vi "graphModule.vi"() -> ()   [LabVIEW 2023]
uses:
  <vilib>/Utility/miscctls.llb/LVCursorListTypeDef.ctl
panel:
  in  "Linked?":bool
  out "gate":i32
  out "Cursor Out":dbl[](array[numeric])=[128.0, 112.0, 144.0, 96.0, 160.0]
  in  "Cursor List":T1=[{"Name"="FGV", "Color"=99999, "Style"=2, "Point Style"=0, "Name Visible"=FALSE, "Allow Drag"=TRUE, "Cursor Mode"=1, "Plot"=0, "Index"=128, "Position"={"X"=128.0, "Y"=0.0}, "X Scale"=0, "Y Scale"=0, "Watch Plots"=[], "Watch All Plots"=FALSE, "Plot Area"=0, "Label Offset"={"X"=0.0, "Y"=0.0}}, {"Name"="Lower Bound", "Color"=50000, "Style"=2, "Point Style"=0, "Name Visible"=FALSE, "Allow Drag"=TRUE, "Cursor Mode"=1, "Plot"=0, "Index"=96, "Position"={"X"=96.0, "Y"=0.0}, "X Scale"=0, "Y Scale"=0, "Watch Plots"=[], "Watch All Plots"=FALSE, "Plot Area"=0, "Label Offset"={"X"=0.0, "Y"=0.0}}, {"Name"="Upper Bound", "Color"=50000, "Style"=2, "Point Style"=0, "Name Visible"=FALSE, "Allow Drag"=TRUE, "Cursor Mode"=1, "Plot"=0, "Index"=160, "Position"={"X"=160.0, "Y"=0.0}, "X Scale"=0, "Y Scale"=0, "Watch Plots"=[], "Watch All Plots"=FALSE, "Plot Area"=0, "Label Offset"={"X"=0.0, "Y"=0.0}}, {"Name"="Int lower", "Color"=16776960, "Style"=2, "Point Style"=0, "Name Visible"=FALSE, "Allow Drag"=TRUE, "Cursor Mode"=1, "Plot"=0, "Index"=80, "Position"={"X"=80.0, "Y"=0.0}, "X Scale"=0, "Y Scale"=0, "Watch Plots"=[], "Watch All Plots"=FALSE, "Plot Area"=0, "Label Offset"={"X"=0.0, "Y"=0.0}}, {"Name"="Int upper", "Color"=16776960, "Style"=2, "Point Style"=0, "Name Visible"=FALSE, "Allow Drag"=TRUE, "Cursor Mode"=1, "Plot"=0, "Index"=176, "Position"={"X"=176.0, "Y"=0.0}, "X Scale"=0, "Y Scale"=0, "Watch Plots"=[], "Watch All Plots"=FALSE, "Plot Area"=0, "Label Offset"={"X"=0.0, "Y"=0.0}}]
  in  "Table Control":bool=TRUE
  in  "Name":string="Gate #"
  out "index":i32
  in  "Cursor Pos":dbl[](array[numeric])=[128.0, 112.0, 144.0, 96.0, 160.0]
  out "Array Waveform":waveform(dbl)(graph)
  # "Gate #"
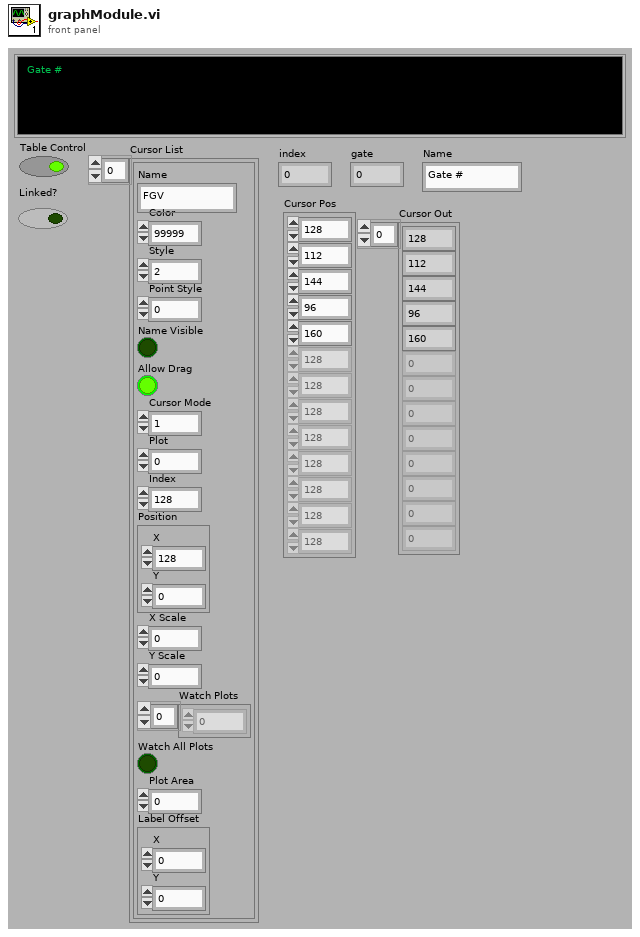
[diagram p1: front panel]
types:
  T1 = typedef "LVCursorListTypeDef.ctl" = cluster{"Name":string, "Color":u32, "Style":u8, "Point Style":u8, "Name Visible":bool, "Allow Drag":bool, "Cursor Mode":u32, "Plot":i32, "Index":i32, "Position":cluster{"X":dbl, "Y":dbl}, "X Scale":u32, "Y Scale":u32, "Watch Plots":i32[], "Watch All Plots":bool, "Plot Area":i32, "Label Offset":cluster{"X":dbl, "Y":dbl}}[]
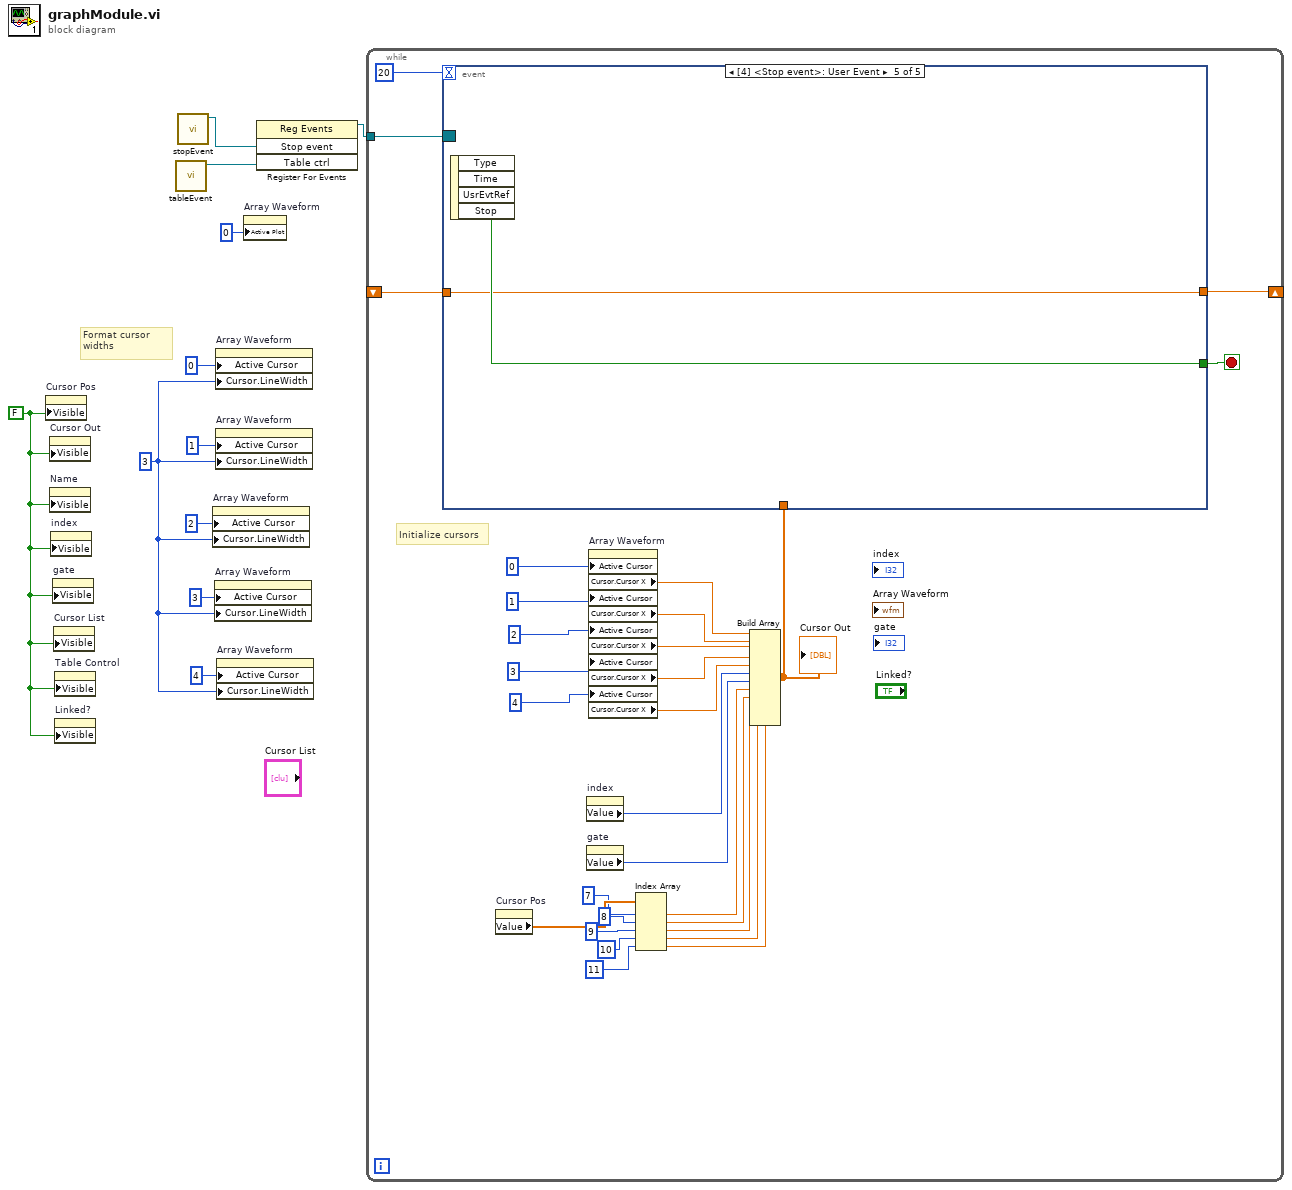
[diagram p0: block diagram]
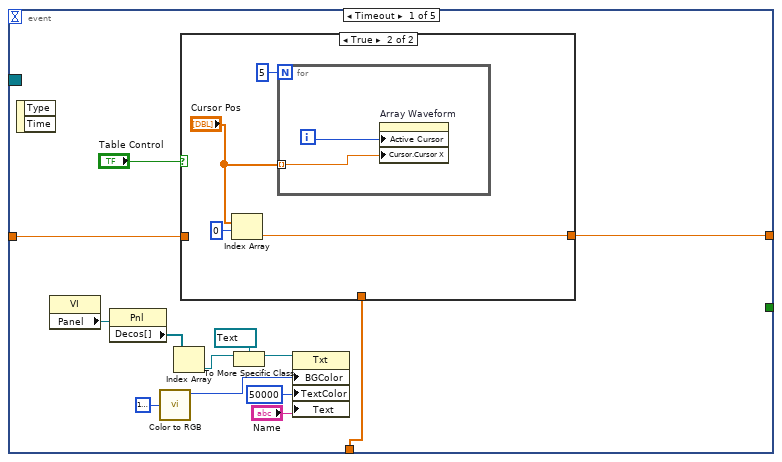
[diagram p2: hidden frame]
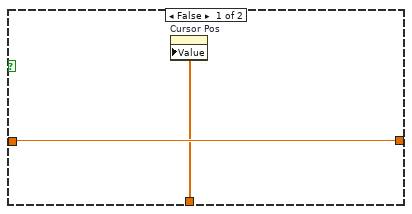
[diagram p3: hidden frame]
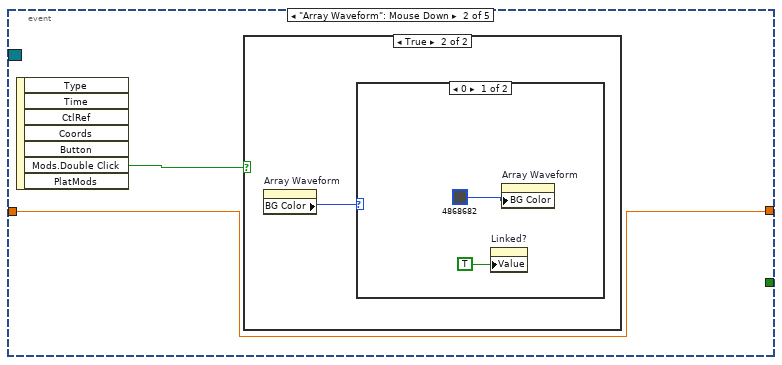
[diagram p4: hidden frame]
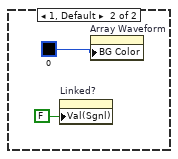
[diagram p6: hidden frame]
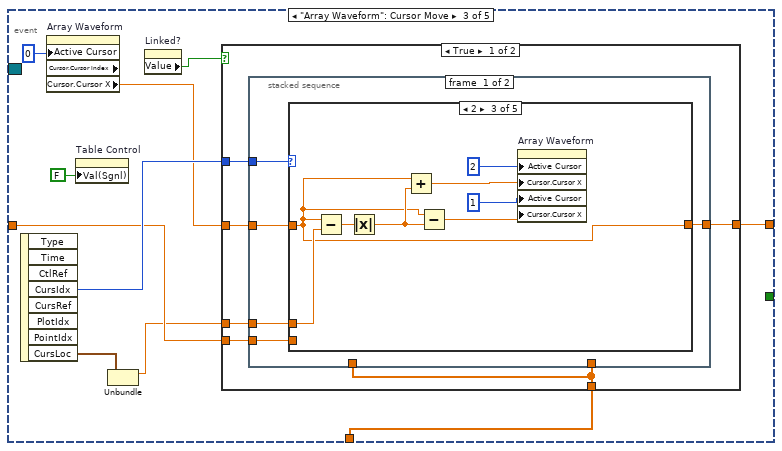
[diagram p7: hidden frame]
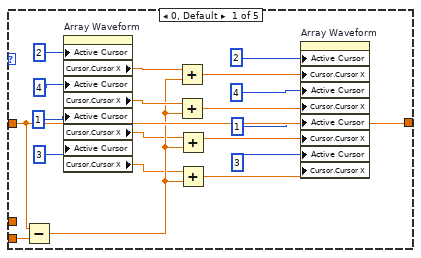
[diagram p8: hidden frame]
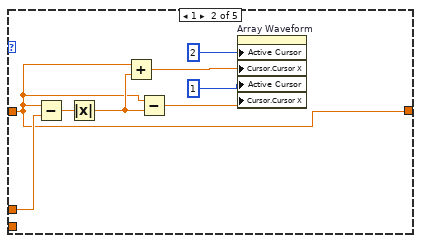
[diagram p9: hidden frame]
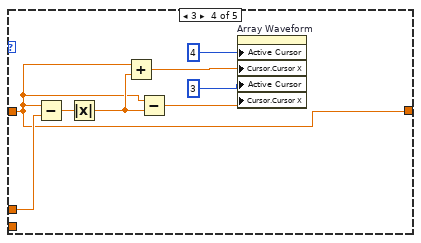
[diagram p10: hidden frame]
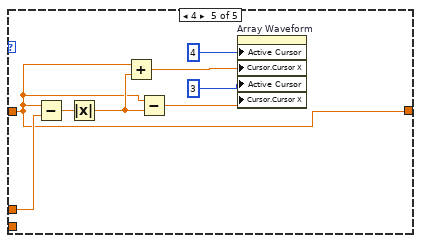
[diagram p11: hidden frame]
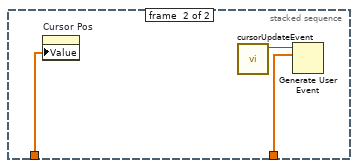
[diagram p12: hidden frame]
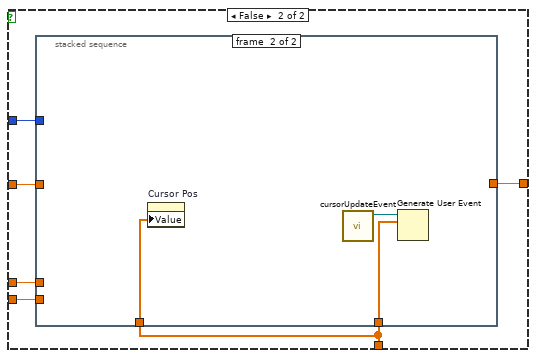
[diagram p13: hidden frame]
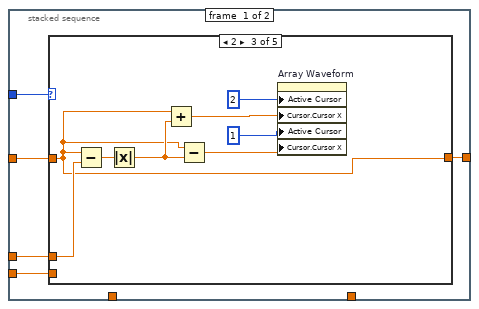
[diagram p14: hidden frame]
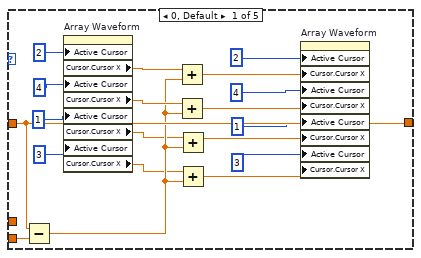
[diagram p15: hidden frame]
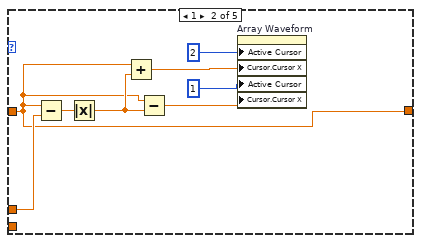
[diagram p16: hidden frame]
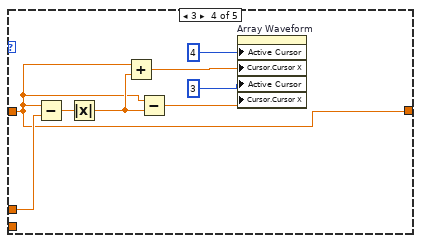
[diagram p17: hidden frame]
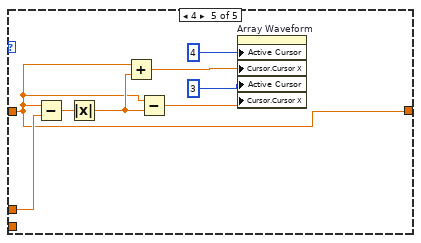
[diagram p18: hidden frame]
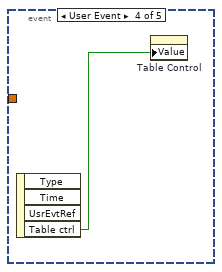
[diagram p19: hidden frame]
diagram:
  w1 = FALSE ("Visible")
  w7 = u8 3 ("Cursor.Line Width")
  # "Format cursor widths"
  n1 = property on="Cursor Pos" class="Arr (strict)"("Visible"=w1) -> ()  [unwired: 2 in, 2 out]
  n2 = property on="Cursor Out" class="Arr (strict)"("Visible"=w1) -> ()  [unwired: 2 in, 2 out]
  n3 = property on="Name" class="Str"("Visible"=w1) -> ()  [unwired: 2 in, 2 out]
  n4 = property on="index" class="DigNum (strict)"("Visible"=w1) -> ()  [unwired: 2 in, 2 out]
  n5 = property on="gate" class="DigNum (strict)"("Visible"=w1) -> ()  [unwired: 2 in, 2 out]
  n6 = property on="Cursor List" class="Arr (strict)"("Visible"=w1) -> ()  [unwired: 2 in, 2 out]
  n7 = property on="Table Control" class="Bool (strict)"("Visible"=w1) -> ()  [unwired: 2 in, 2 out]
  n8 = property on="Linked?" class="Bool (strict)"("Visible"=w1) -> ()  [unwired: 2 in, 2 out]
  n9 = call "tableEvent.vi"() -> ("Table ctrl"=w2:refnum<user-event>)  [unwired: 11 in]
  n10 = call "stopEvent.vi"() -> ("Stop event"=w4:refnum<user-event>)  [unwired: 11 out]
  n11 = property on="Array Waveform" class="WFGraph (strict)"("Active Cursor"=u32 2, "Cursor.LineWidth"=w7) -> ()  [unwired: 2 in, 2 out]
  n12 = property on="Array Waveform" class="WFGraph (strict)"("Active Cursor"=u32 3, "Cursor.LineWidth"=w7) -> ()  [unwired: 2 in, 2 out]
  n13 = property on="Array Waveform" class="WFGraph (strict)"("Active Cursor"=u32 0, "Cursor.LineWidth"=w7) -> ()  [unwired: 2 in, 2 out]
  n14 = property on="Array Waveform" class="WFGraph (strict)"("Active Cursor"=u32 1, "Cursor.LineWidth"=w7) -> ()  [unwired: 2 in, 2 out]
  n15 = property on="Array Waveform" class="WFGraph (strict)"("Active Cursor"=u32 4, "Cursor.LineWidth"=w7) -> ()  [unwired: 2 in, 2 out]
  n16 = property on="Array Waveform" class="WFGraph (strict)"("Active Plot"=u32 0) -> ()  [unwired: 2 in, 2 out]
  n17 = register-events(w4, w2) -> (reference out=w11:refnum<event-registration>)  [unwired: 2 in, 1 out]
  n18 = while {
    tunnel: w11 -> [w40]
    shift-right: [w37] -> _
    shift-left: _ -> [w38]
    stop <- w39 stop-if-true
    # "Initialize cursors"
    n19 = property on="Cursor Pos" class="Arr (strict)"() -> ("Value"=w22:dbl[])  [unwired: 2 in, 2 out]
    n20 = property on="index" class="DigNum (strict)"() -> ("Value"=w25:i32)  [unwired: 2 in, 2 out]
    n21 = property on="gate" class="DigNum (strict)"() -> ("Value"=w24:i32)  [unwired: 2 in, 2 out]
    n22 = property on="Array Waveform" class="WFGraph (strict)"("Active Cursor"=u32 0, "Active Cursor"=u32 1, "Active Cursor"=u32 2, "Active Cursor"=u32 3, "Active Cursor"=u32 4) -> ("Cursor.Cursor X"=w35:dbl, "Cursor.Cursor X"=w32:dbl, "Cursor.Cursor X"=w34:dbl, "Cursor.Cursor X"=w33:dbl, "Cursor.Cursor X"=w31:dbl)  [unwired: 2 in, 2 out]
    n23 = Index Array(array=w22, index #1=7 ("index"), index #2=8 ("index"), index #3=9 ("index"), index #4=10 ("index"), index #5=11 ("index")) -> (element #1=w16:dbl, element #2=w15:dbl, element #3=w14:dbl, element #4=w13:dbl, element #5=w12:dbl)
    n24 = Build Array(w35, w32, w34, w33, w31, w25, w24, w16, w15, w14, w13, w12) -> (w23:dbl[])
    "Cursor Out" <- w23
    n25 = event shown="[4] <Stop event>: User Event" {
      selector: w40 -> [_ _ _ _ _]
      dyn-events: _ -> [_ _ _ _ _]
      timeout: 20 -> [_ _ _ _ _]
      tunnel: [_ _ _ _ w211] -> w39
      tunnel: w38 -> [w42 w62 w77 _ w210]
      tunnel: [w43 w62 w76 _ w210] -> w37
      tunnel: w23 -> [w41 _ w72 _ _]
      event Timeout {
        n26 = event-data() -> ()  [unwired: 1 in, 2 out]
        n27 = property class="VI"() -> ("Panel"=w51:refnum<vi>)  [unwired: 2 in, 2 out]
        n28 = property class="Pnl"(reference=w51) -> ("Decos[]"=w49:refnum<vi>[])  [unwired: 1 in, 2 out]
        n29 = call <vilib>:"Color to RGB.vi"("Color"=u32 16777216) -> ("Resolved Color"=w53:u32)  [unwired: 3 out]
        n30 = Index Array(array=w49) -> (element=w48:refnum<vi>)  [unwired: 1 in]
        n31 = case shown="True" "Table Control" {
          tunnel: [w55 w58] -> w43
          tunnel: w42 -> [w55 _]
          tunnel: w41 -> [w54 _]
          frame False {
            n32 = property on="Cursor Pos" class="Arr (strict)"("Value"=w54) -> ()  [unwired: 2 in, 2 out]
          }
          frame True {
            n33 = Index Array(array="Cursor Pos", index=0) -> (element=w58:dbl)
            n34 = for {
              N: 5 -> [_]
              tunnel: "Cursor Pos" -> [w60] mode=indexing
              i -> [w61]
              n35 = property on="Array Waveform" class="WFGraph (strict)"("Active Cursor"=w61, "Cursor.Cursor X"=w60) -> ()  [unwired: 2 in, 2 out]
            }
          }
        }
        n36 = To More Specific Class(target class=refnum<vi> refnum, reference=w48) -> (specific class reference=w47:refnum<vi>)  [unwired: 1 in, 1 out]
        n37 = property class="Txt"(reference=w47, "BGColor"=w53, "TextColor"=u32 50000 ("Text Colors:Text Color"), "Text"="Name") -> ()  [unwired: 1 in, 2 out]
      }
      event "Array Waveform": Mouse Down {
        n38 = event-data() -> ("Mods.Double Click"=w63:bool)  [unwired: 1 in, 6 out]
        n39 = case shown="True" w63 {
          frame False {
          }
          frame True {
            n40 = property on="Array Waveform" class="WFGraph (strict)"() -> ("BG Color"=w64:u32)  [unwired: 2 in, 2 out]
            n41 = case shown="0" w64 {
              frame 0 {
                n42 = property on="Linked?" class="Bool (strict)"("Value"=TRUE ("Value (Signaling)")) -> ()  [unwired: 2 in, 2 out]
                n43 = property on="Array Waveform" class="WFGraph (strict)"("BG Color"=u32 4868682) -> ()  [unwired: 2 in, 2 out]
              }
              frame 1, Default {
                n44 = property on="Linked?" class="Bool (strict)"("Val(Sgnl)"=FALSE ("Value (Signaling)")) -> ()  [unwired: 2 in, 2 out]
                n45 = property on="Array Waveform" class="WFGraph (strict)"("BG Color"=u32 0) -> ()  [unwired: 2 in, 2 out]
              }
            }
          }
        }
      }
      event "Array Waveform": Cursor Move {
        n46 = event-data() -> ("CursIdx"=w78:i32, "CursLoc"=w71:cluster{"X":dbl, "Y":dbl})  [unwired: 1 in, 6 out]
        n47 = property on="Array Waveform" class="WFGraph (strict)" props=["Active Cursor", "Cursor", "Cursor Index", "Cursor", "Cursor X"]("Active Cursor"=u32 0) -> ("Cursor.Cursor X"=w73:dbl)  [unwired: 2 in, 3 out]
        n48 = property on="Table Control" class="Bool (strict)"("Val(Sgnl)"=FALSE ("Value (Signaling)")) -> ()  [unwired: 2 in, 2 out]
        n49 = Unbundle(w71) -> ("X"=w70:dbl)  [unwired: 1 out]
        n50 = property on="Linked?" class="Bool (strict)"() -> ("Value"=w69:bool)  [unwired: 2 in, 2 out]
        n51 = case shown="True" w69 {
          tunnel: w78 -> [w84 w149]
          tunnel: w77 -> [w83 w148]
          tunnel: [w82 w147] -> w76
          tunnel: w73 -> [w81 w146]
          tunnel: w72 -> [w80 w145]
          tunnel: w70 -> [w79 w144]
          frame True {
            n52 = stacked-sequence {
              tunnel: w84 -> [w89 _]
              tunnel: w83 -> [w88 _]
              tunnel: [w87 _] -> w82
              tunnel: w79 -> [w86 _]
              tunnel: w81 -> [w85 _]
              tunnel: w80 -> [_ w142]
              tunnel: w80 -> [_ w141]
              frame #0 {
                n53 = case shown="2" w89 {
                  tunnel: w85 -> [w106 w111 w119 w127 w135]
                  tunnel: w86 -> [_ w116 w124 w132 w140]
                  tunnel: [w106 w111 w119 w127 w135] -> w87
                  tunnel: w88 -> [w105 _ _ _ _]
                  frame 0, Default {
                    n54 = Subtract(x=w106, y=w105) -> (x-y=w101:dbl)
                    n55 = property on="Array Waveform" class="WFGraph (strict)"("Active Cursor"=u32 2, "Active Cursor"=u32 4, "Active Cursor"=u32 1, "Active Cursor"=u32 3) -> ("Cursor.Cursor X"=w104:dbl, "Cursor.Cursor X"=w102:dbl, "Cursor.Cursor X"=w93:dbl, "Cursor.Cursor X"=w92:dbl)  [unwired: 2 in, 2 out]
                    n56 = Add(x=w104, y=w101) -> (x+y=w103:dbl)
                    n57 = Add(x=w102, y=w101) -> (x+y=w99:dbl)
                    n58 = Add(x=w93, y=w101) -> (x+y=w96:dbl)
                    n59 = Add(x=w92, y=w101) -> (x+y=w94:dbl)
                    n60 = property on="Array Waveform" class="WFGraph (strict)"("Active Cursor"=u32 2, "Cursor.Cursor X"=w103, "Active Cursor"=u32 4, "Cursor.Cursor X"=w99, "Active Cursor"=u32 1, "Cursor.Cursor X"=w96, "Active Cursor"=u32 3, "Cursor.Cursor X"=w94) -> ()  [unwired: 2 in, 2 out]
                  }
                  frame 1 {
                    n61 = Subtract(x=w111, y=w116) -> (x-y=w114:dbl)
                    n62 = Absolute Value(x=w114) -> (abs(x)=w112:dbl)
                    n63 = Add(x=w111, y=w112) -> (x+y=w113:dbl)
                    n64 = Subtract(x=w111, y=w112) -> (x-y=w109:dbl)
                    n65 = property on="Array Waveform" class="WFGraph (strict)"("Active Cursor"=u32 2, "Cursor.Cursor X"=w113, "Active Cursor"=u32 1, "Cursor.Cursor X"=w109) -> ()  [unwired: 2 in, 2 out]
                  }
                  frame 2 {
                    n66 = Subtract(x=w119, y=w124) -> (x-y=w122:dbl)
                    n67 = Absolute Value(x=w122) -> (abs(x)=w120:dbl)
                    n68 = Add(x=w119, y=w120) -> (x+y=w121:dbl)
                    n69 = Subtract(x=w119, y=w120) -> (x-y=w117:dbl)
                    n70 = property on="Array Waveform" class="WFGraph (strict)"("Active Cursor"=u32 2, "Cursor.Cursor X"=w121, "Active Cursor"=u32 1, "Cursor.Cursor X"=w117) -> ()  [unwired: 2 in, 2 out]
                  }
                  frame 3 {
                    n71 = Subtract(x=w127, y=w132) -> (x-y=w130:dbl)
                    n72 = Absolute Value(x=w130) -> (abs(x)=w128:dbl)
                    n73 = Add(x=w127, y=w128) -> (x+y=w129:dbl)
                    n74 = Subtract(x=w127, y=w128) -> (x-y=w125:dbl)
                    n75 = property on="Array Waveform" class="WFGraph (strict)"("Active Cursor"=u32 4, "Cursor.Cursor X"=w129, "Active Cursor"=u32 3, "Cursor.Cursor X"=w125) -> ()  [unwired: 2 in, 2 out]
                  }
                  frame 4 {
                    n76 = Subtract(x=w135, y=w140) -> (x-y=w138:dbl)
                    n77 = Absolute Value(x=w138) -> (abs(x)=w136:dbl)
                    n78 = Add(x=w135, y=w136) -> (x+y=w137:dbl)
                    n79 = Subtract(x=w135, y=w136) -> (x-y=w133:dbl)
                    n80 = property on="Array Waveform" class="WFGraph (strict)"("Active Cursor"=u32 4, "Cursor.Cursor X"=w137, "Active Cursor"=u32 3, "Cursor.Cursor X"=w133) -> ()  [unwired: 2 in, 2 out]
                  }
                }
              }
              frame #1 {
                n81 = property on="Cursor Pos" class="Arr (strict)"("Value"=w141) -> ()  [unwired: 2 in, 2 out]
                n82 = call "cursorUpdateEvent.vi"() -> ("Cursor Array"=w143:refnum<user-event>)  [unwired: 11 in]
                n83 = Generate User Event(user event=w143, event data cluster=w142) -> ()  [unwired: 2 in, 2 out]
              }
            }
          }
          frame False {
            n84 = stacked-sequence {
              tunnel: w149 -> [w154 _]
              tunnel: w148 -> [w153 _]
              tunnel: [w152 _] -> w147
              tunnel: w144 -> [w151 _]
              tunnel: w146 -> [w150 _]
              tunnel: w145 -> [_ w207]
              tunnel: w145 -> [_ w206]
              frame #0 {
                n85 = case shown="2" w154 {
                  tunnel: w150 -> [w171 w176 w184 w192 w200]
                  tunnel: w151 -> [_ w181 w189 w197 w205]
                  tunnel: [w171 w176 w184 w192 w200] -> w152
                  tunnel: w153 -> [w170 _ _ _ _]
                  frame 0, Default {
                    n86 = Subtract(x=w171, y=w170) -> (x-y=w166:dbl)
                    n87 = property on="Array Waveform" class="WFGraph (strict)"("Active Cursor"=u32 2, "Active Cursor"=u32 4, "Active Cursor"=u32 1, "Active Cursor"=u32 3) -> ("Cursor.Cursor X"=w169:dbl, "Cursor.Cursor X"=w167:dbl, "Cursor.Cursor X"=w158:dbl, "Cursor.Cursor X"=w157:dbl)  [unwired: 2 in, 2 out]
                    n88 = Add(x=w169, y=w166) -> (x+y=w168:dbl)
                    n89 = Add(x=w167, y=w166) -> (x+y=w164:dbl)
                    n90 = Add(x=w158, y=w166) -> (x+y=w161:dbl)
                    n91 = Add(x=w157, y=w166) -> (x+y=w159:dbl)
                    n92 = property on="Array Waveform" class="WFGraph (strict)"("Active Cursor"=u32 2, "Cursor.Cursor X"=w168, "Active Cursor"=u32 4, "Cursor.Cursor X"=w164, "Active Cursor"=u32 1, "Cursor.Cursor X"=w161, "Active Cursor"=u32 3, "Cursor.Cursor X"=w159) -> ()  [unwired: 2 in, 2 out]
                  }
                  frame 1 {
                    n93 = Subtract(x=w176, y=w181) -> (x-y=w179:dbl)
                    n94 = Absolute Value(x=w179) -> (abs(x)=w177:dbl)
                    n95 = Add(x=w176, y=w177) -> (x+y=w178:dbl)
                    n96 = Subtract(x=w176, y=w177) -> (x-y=w174:dbl)
                    n97 = property on="Array Waveform" class="WFGraph (strict)"("Active Cursor"=u32 2, "Cursor.Cursor X"=w178, "Active Cursor"=u32 1, "Cursor.Cursor X"=w174) -> ()  [unwired: 2 in, 2 out]
                  }
                  frame 2 {
                    n98 = Subtract(x=w184, y=w189) -> (x-y=w187:dbl)
                    n99 = Absolute Value(x=w187) -> (abs(x)=w185:dbl)
                    n100 = Add(x=w184, y=w185) -> (x+y=w186:dbl)
                    n101 = Subtract(x=w184, y=w185) -> (x-y=w182:dbl)
                    n102 = property on="Array Waveform" class="WFGraph (strict)"("Active Cursor"=u32 2, "Cursor.Cursor X"=w186, "Active Cursor"=u32 1, "Cursor.Cursor X"=w182) -> ()  [unwired: 2 in, 2 out]
                  }
                  frame 3 {
                    n103 = Subtract(x=w192, y=w197) -> (x-y=w195:dbl)
                    n104 = Absolute Value(x=w195) -> (abs(x)=w193:dbl)
                    n105 = Add(x=w192, y=w193) -> (x+y=w194:dbl)
                    n106 = Subtract(x=w192, y=w193) -> (x-y=w190:dbl)
                    n107 = property on="Array Waveform" class="WFGraph (strict)"("Active Cursor"=u32 4, "Cursor.Cursor X"=w194, "Active Cursor"=u32 3, "Cursor.Cursor X"=w190) -> ()  [unwired: 2 in, 2 out]
                  }
                  frame 4 {
                    n108 = Subtract(x=w200, y=w205) -> (x-y=w203:dbl)
                    n109 = Absolute Value(x=w203) -> (abs(x)=w201:dbl)
                    n110 = Add(x=w200, y=w201) -> (x+y=w202:dbl)
                    n111 = Subtract(x=w200, y=w201) -> (x-y=w198:dbl)
                    n112 = property on="Array Waveform" class="WFGraph (strict)"("Active Cursor"=u32 4, "Cursor.Cursor X"=w202, "Active Cursor"=u32 3, "Cursor.Cursor X"=w198) -> ()  [unwired: 2 in, 2 out]
                  }
                }
              }
              frame #1 {
                n113 = property on="Cursor Pos" class="Arr (strict)"("Value"=w206) -> ()  [unwired: 2 in, 2 out]
                n114 = call "cursorUpdateEvent.vi"() -> ("Cursor Array"=w208:refnum<user-event>)  [unwired: 11 in]
                n115 = Generate User Event(user event=w208, event data cluster=w207) -> ()  [unwired: 2 in, 2 out]
              }
            }
          }
        }
      }
      event User Event {
        n116 = event-data() -> ("Table ctrl"=w209:bool)  [unwired: 1 in, 3 out]
        n117 = property on="Table Control" class="Bool (strict)"("Value"=w209) -> ()  [unwired: 2 in, 2 out]
      }
      event User Event {
        n118 = event-data() -> ("Stop"=w211:bool)  [unwired: 1 in, 3 out]
      }
    }
  }
